vi "ServerAsControllerEXP.vi"() -> ()   [LabVIEW 2020]
panel:
  out "d":dbl[](array[numeric])
  out "CP Heat":dbl[](array[numeric])
  out "CSV Time":dbl[](array[numeric])
  out "x0":dbl[](array[numeric])
  out "Predicted States":dbl[](array[numeric])
  out "Length of states":i32
  out "data size":i32
  out "k":dbl
  out "Measured States":dbl[](array[numeric])
  in  "stop":bool
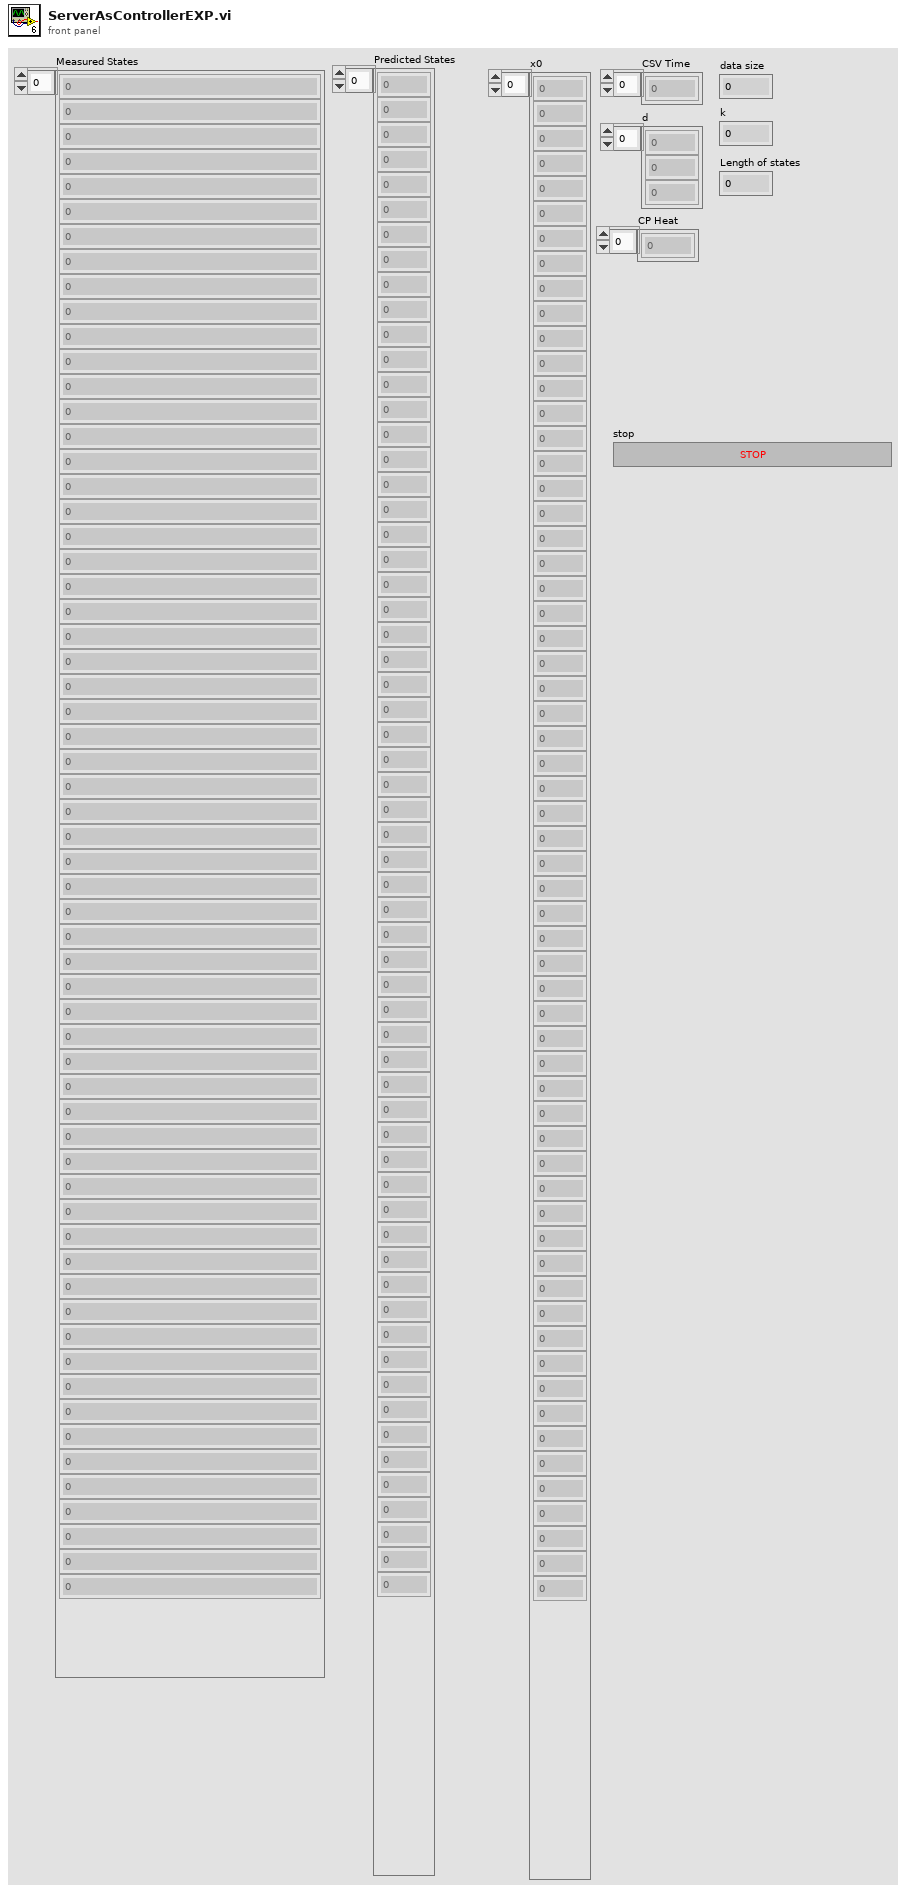
[diagram p1: front panel]
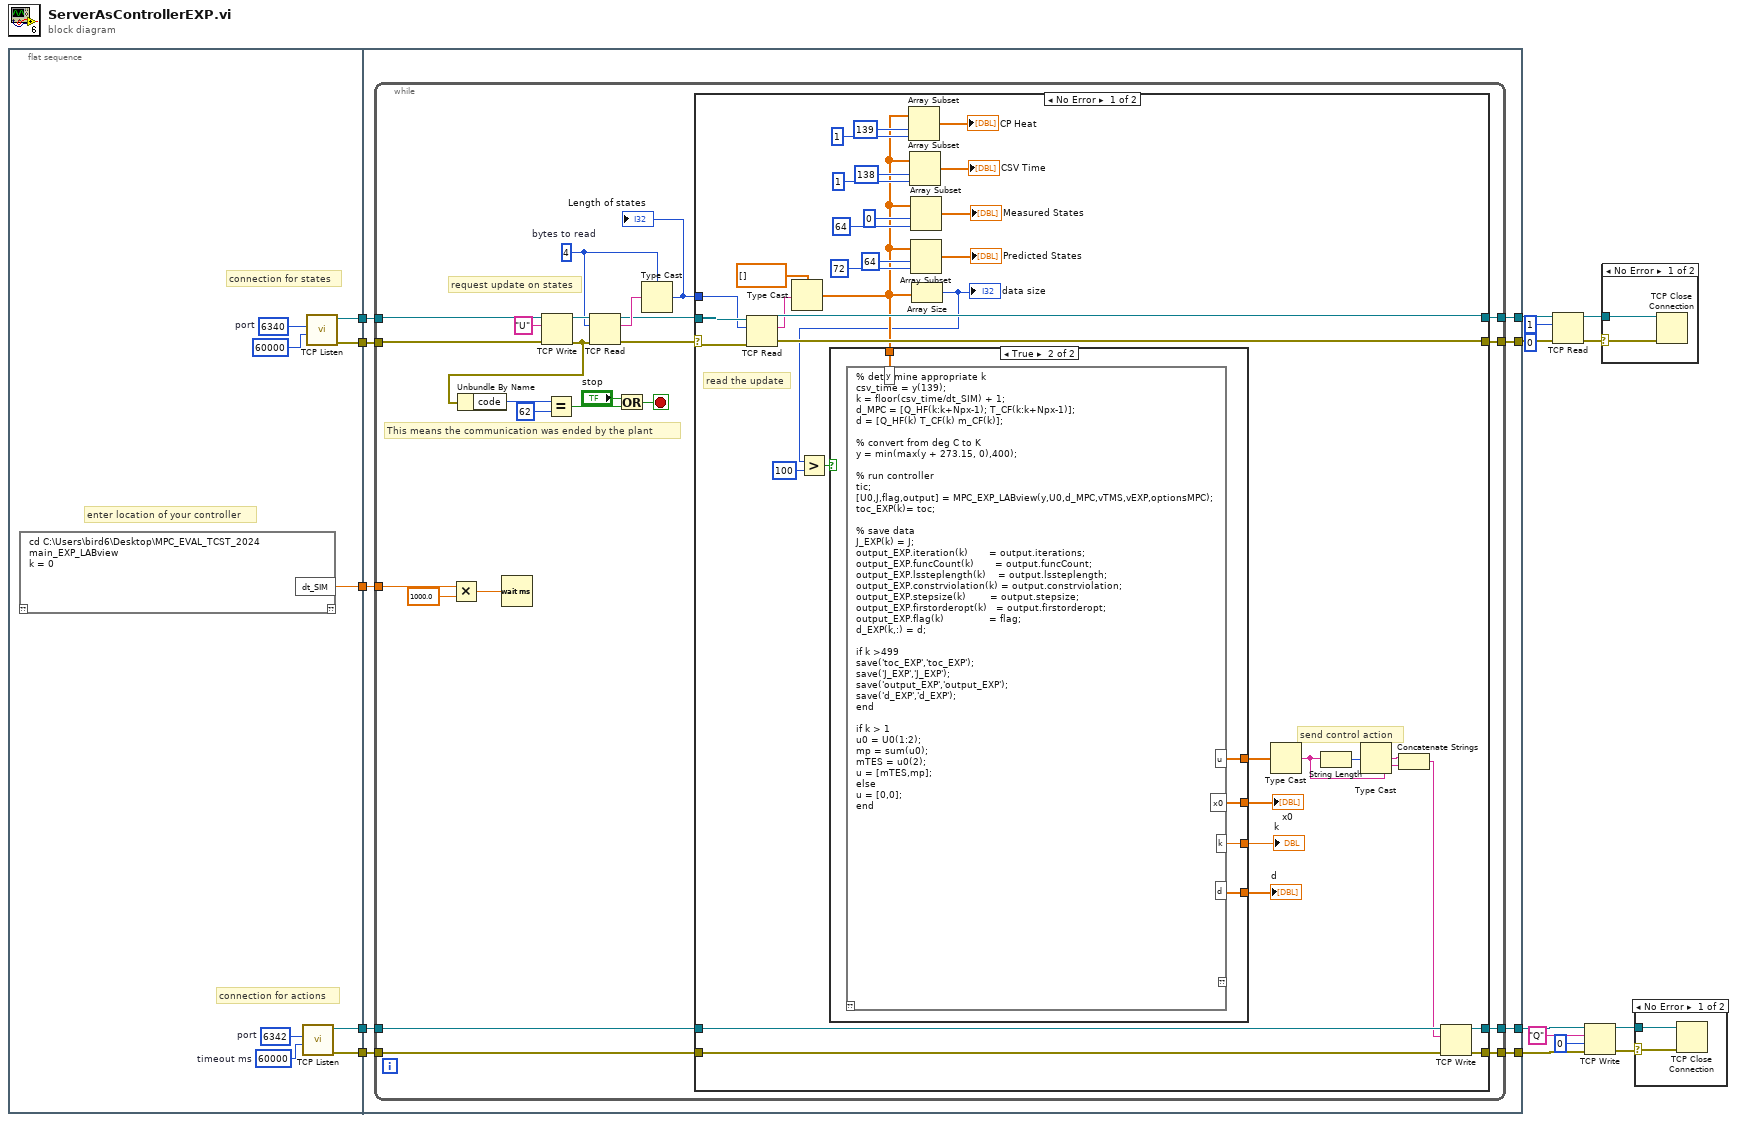
[diagram p0: block diagram]
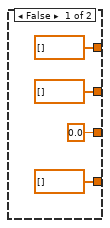
[diagram p4: hidden frame]
diagram:
  n1 = flat-sequence {
    tunnel: [w23] -> w17
    tunnel: [w22] -> w16
    tunnel: [w21] -> w15
    tunnel: [w20] -> w14
    tunnel: [w19] -> w2
    tunnel: w17 -> [w31]
    tunnel: w16 -> [w30]
    tunnel: w15 -> [w29]
    tunnel: w14 -> [w28]
    tunnel: w2 -> [w27]
    tunnel: [w35] -> w13
    tunnel: [w34] -> w12
    tunnel: [w33] -> w10
    tunnel: [w32] -> w9
    frame #0 {
      w25 = u16 6342  # port
      w26 = 60000  # timeout ms
      w24 = u16 6340  # port
      # "enter location of your controller"
      # "connection for actions"
      # "connection for states"
      n2 = script code="cd C:\\Users\\bird6\\Desktop\\MPC_EVAL_TCST_2024\nmain_EXP_LABview\nk = 0"() -> ("dt_SIM"=w19:dbl)  [unwired: 1 in, 1 out]
      n3 = call <vilib>:"TCP Listen.vi"("timeout ms (wait forever: -1)"=w26, "port"=w25) -> ("error out"=w23:errorcluster, "connection ID"=w22:refnum<k5>)  [unwired: 5 in, 3 out]
      n4 = call <vilib>:"TCP Listen.vi"("timeout ms (wait forever: -1)"=60000, "port"=w24) -> ("error out"=w21:errorcluster, "connection ID"=w20:refnum<k5>)  [unwired: 5 in, 3 out]
    }
    frame #1 {
      n5 = while {
        tunnel: [w59] -> w35
        tunnel: [w58] -> w34
        tunnel: [w57] -> w33
        tunnel: [w56] -> w32
        tunnel: w31 -> [w52]
        tunnel: w30 -> [w55]
        tunnel: w29 -> [w54]
        tunnel: w28 -> [w53]
        tunnel: w27 -> [w38]
        stop <- w39 stop-if-true
        w46 = 4  # bytes to read
        # "This means the communication was ended by the plant"
        # "request update on states"
        n6 = Multiply(x=w38, y=1000.0) -> (x*y=w36:dbl)
        n7 = Wait (ms)(milliseconds to wait=w36) -> ()  [unwired: 1 out]
        n8 = TCP Write(connection ID=w53, data in="U", error in (no error)=w54) -> (connection ID out=w49:refnum<k5>, error out=w44:errorcluster)  [unwired: 2 out]
        n9 = Unbundle By Name(w44) -> ("code"=w43:i32)
        n10 = Equal?(x=w43, y=62) -> (x = y?=w40:bool)
        n11 = TCP Read(connection ID=w49, bytes to read=w46, error in (no error)=w44) -> (connection ID out=w47:refnum<k5>, data out=w50:string, error out=w45:errorcluster)  [unwired: 2 in]
        n12 = Or(x="stop", y=w40) -> (x .or. y?=w39:bool)
        n13 = Type Cast(type=w46, x=w50) -> (*(type *) &x=w48:i32)
        "Length of states" <- w48
        n14 = case shown="No Error" w45 {
          selector: w45 -> [w86 w104]
          tunnel: [w94 w107] -> w59
          tunnel: [w93 w104] -> w58
          tunnel: [w92 w106] -> w57
          tunnel: [w91 w105] -> w56
          tunnel: w55 -> [w85 w106]
          tunnel: w52 -> [w84 w105]
          tunnel: w48 -> [w68 _]
          tunnel: w47 -> [w90 w107]
          frame No Error {
            # "send control action"
            # "read the update"
            n15 = TCP Read(connection ID=w90, bytes to read=w68, error in (no error)=w86) -> (connection ID out=w94:refnum<k5>, data out=w89:string, error out=w93:errorcluster)  [unwired: 2 in]
            n16 = Type Cast(type=dbl[] [], x=w89) -> (*(type *) &x=w67:dbl[])
            n17 = Array Subset(array=w67, index=139, length=1) -> (→"CP Heat":dbl[])
            n18 = Array Subset(array=w67, index=138, length=1) -> (→"CSV Time":dbl[])
            n19 = Array Subset(array=w67, index=0, length=64) -> (→"Measured States":dbl[])
            n20 = Array Subset(array=w67, index=64, length=72) -> (→"Predicted States":dbl[])
            n21 = Array Size(array=w67) -> (size(s)=w61:i32)
            "data size" <- w61
            n22 = Greater?(x=w61, y=100) -> (0:w62:bool)
            n23 = case shown="True" w62 {
              tunnel: w67 -> [_ w103]
              tunnel: [dbl[] [] w102] -> w66
              tunnel: [0.0 w101] -> w65
              tunnel: [dbl[] [] w100] -> w64
              tunnel: [dbl[] [] w99] -> w63
              frame False {
              }
              frame True {
                # "Compute control action"
                n24 = script code="% determine appropriate k\ncsv_time = y(139);\nk = floor(csv_time/dt_SIM) + 1;\nd_MPC = [Q_HF(k:k+Npx-1); T_CF(k:k+Npx-1)];\nd = [Q_HF(k) T_CF(k) m_CF(k)];\n\n% convert from deg C to K\ny = min(max(y + 273.15, 0),400);\n\n% run controller\ntic;\n[U0,J,flag,output] = MPC_EXP_LABview(y,U0,d_MPC,vTMS,vEXP,optionsMPC);\ntoc_EXP(k)= toc;\n\n% save data\nJ_EXP(k) = J;\noutput_EXP.iteration(k)       = output.iterations;\noutput_EXP.funcCount(k)       = output.funcCount;\noutput_EXP.lssteplength(k)    = output.lssteplength;\noutput_EXP.constrviolation(k) = output.constrviolation;\noutput_EXP.stepsize(k)        = output.stepsize;\noutput_EXP.firstorderopt(k)   = output.firstorderopt;\noutput_EXP.flag(k)               = flag;\nd_EXP(k,:) = d;\n\nif k >499\nsave('toc_EXP','toc_EXP');\nsave('J_EXP','J_EXP');\nsave('output_EXP','output_EXP');\nsave('d_EXP','d_EXP');\nend\n\nif k > 1\nu0 = U0(1:2);\nmp = sum(u0);\nmTES = u0(2);\nu = [mTES,mp];\nelse\nu = [0,0];\nend"("y"=w103) -> ("u"=w102:dbl[], "k"=w101:dbl, "x0"=w100:dbl[], "d"=w99:dbl[])  [unwired: 1 in, 1 out]
              }
            }
            "k" <- w65
            "x0" <- w64
            "d" <- w63
            n25 = Type Cast(x=w66) -> (*(type *) &x=w81:string)  [unwired: 1 in]
            n26 = String Length(string=w81) -> (length=w87:i32)
            n27 = Type Cast(x=w87) -> (*(type *) &x=w82:string)  [unwired: 1 out]
            n28 = Concatenate Strings(w82, w81) -> (w83:string)
            n29 = TCP Write(connection ID=w85, data in=w83, error in (no error)=w84) -> (connection ID out=w92:refnum<k5>, error out=w91:errorcluster)  [unwired: 2 out]
          }
          frame Error {
          }
        }
      }
    }
  }
  n30 = TCP Read(connection ID=w13, bytes to read=1, error in (no error)=w12, 9:0 ("timeout ms (25000)")) -> (connection ID out=w6:refnum<k5>, error out=w7:errorcluster)  [unwired: 1 in, 1 out]
  n31 = TCP Write(connection ID=w10, data in="Q", error in (no error)=w9, 9:0 ("timeout ms (25000)")) -> (connection ID out=w5:refnum<k5>, error out=w1:errorcluster)  [unwired: 1 out]
  n32 = case shown="No Error" w7 {
    selector: w7 -> [w108 _]
    tunnel: w6 -> [w109 _]
    frame No Error {
      n33 = TCP Close Connection(connection ID=w109, error in (no error)=w108) -> ()  [unwired: 3 out]
    }
    frame Error {
    }
  }
  n34 = case shown="No Error" w1 {
    selector: w1 -> [w110 _]
    tunnel: w5 -> [w111 _]
    frame No Error {
      n35 = TCP Close Connection(connection ID=w111, error in (no error)=w110) -> ()  [unwired: 3 out]
    }
    frame Error {
    }
  }
